vi "PH_uOPA_DelayController.set Control Status.vi"(0 "VI in":refnum<vi>, 2 "Control Status":T1, 5 "error in (no error)":errorcluster) -> (14 "VI out":refnum<vi>, 19 "error out":errorcluster)   [LabVIEW 2014, in "PH_uOPA_DelayController.lvlib"]
uses:
  PH_uOPA_DelayController.lvlib
  PH_uOPA_DelayController.Control Status.ctl
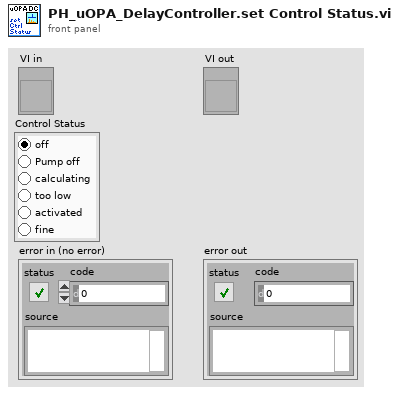
[diagram p1: front panel]
types:
  T1 = typedef "PH_uOPA_DelayController.lvlib/PH_uOPA_DelayController.Control Status.ctl" = enum32{"off", "Pump off", "calculating", "too low", "activated", "fine"}
  T2 = typedef "PH_uOPA_DelayController.lvlib/PH_uOPA_DelayController.i attribute.ctl" = cluster{"GUI Refs":cluster{"Current Pump Peak":refnum<vi>, "Current uOPA Peak":refnum<vi>, "Pump Peak":refnum<vi>, "uOPA Peak":refnum<vi>, "uOPA Target":refnum<vi>, "uOPA Limits [%]":refnum<vi>, "sample length":refnum<vi>, "Pump Target":refnum<vi>, "Pump Limit":refnum<vi>, "Pump running":refnum<vi>, "Feedback Control":refnum<vi>, "Control Status":refnum<vi>, "uOPA Mean":refnum<vi>, "Current uOPA Mean":refnum<vi>}, "uOPA Target":dbl, "uOPA Limits [%]":T3, "Sample Length":i32, "Initialize Mean":bool, "Pump Target":dbl, "Pump Limit [%]":dbl, "Feedback Control":bool, "Control Status":T1, "last Mean":dbl, "last direction":T4, "Axis Settings":T5, "Width while feedback":dbl}
  T3 = typedef "PH_uOPA_DelayController.lvlib/PH_uOPA_DelayController.Limit.ctl" = cluster{"low":dbl, "activate":dbl, "fine":dbl}
  T4 = typedef "PH_Stepmotor_BaseClass.lvlib/PH_Stepmotor_BaseClass.Axis Direction.ctl" = enum16{"forward", "backward"}
  T5 = typedef "PH_Stepmotor_BaseClass.lvlib/PH_Stepmotor_BaseClass.Axis Settings.ctl" = cluster{"Sign change":bool, "Width":dbl, "Calibration":dbl, "Unit":string, "Motor Type":T6, "Unit Width":string, "Unit CF":string}
  T6 = typedef "PH_Stepmotor_BaseClass.lvlib/PH_Stepmotor_BaseClass.Motor Type.ctl" = enum16{"Unspecific", "OWIS 49.120.2633", "OWIS 49.060.1033", "OWIS 43.040.2558", "Diamond Motion 2200 series", "OWIS 49.120.266B.MV6", "Calorimeter", "Linear Stage 1", "MICOS VT-80", "MICOS VT-80 S", "Standa Rotstage nt0.95A", "PUF RA 320.200", "PUF RA 800.200", "PUF RA 800.400", "PUF RA 400.50", "1324.nn.800.50", "1324.n9c.800.50", "1324.nn.320.200", "1324.nn.400.200", "1324.nn.800.200", "1324.nn.400.50", "1324.8c9c.800.50", "1324.8c9c.400.200"}
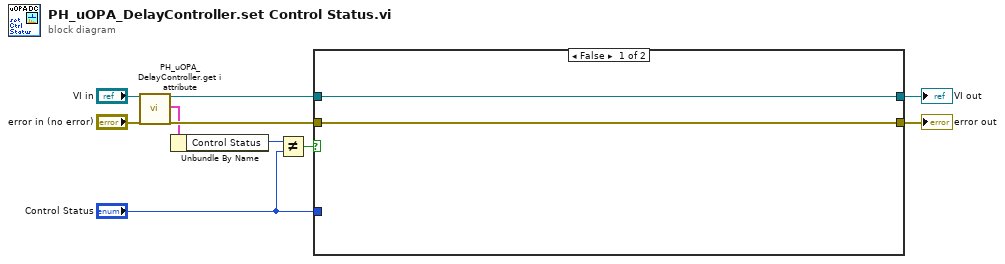
[diagram p0: block diagram]
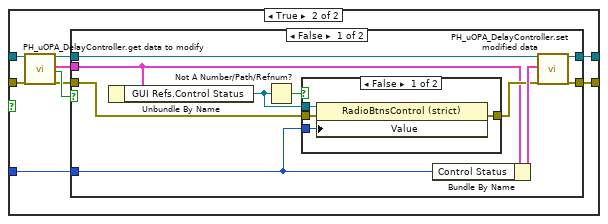
[diagram p2: hidden frame]
diagram:
  n1 = call "PH_uOPA_DelayController.get i attribute.vi"("i ref in"="VI in", "error in (no error)"="error in (no error)") -> ("i ref out"=w5:refnum<vi>, "i attribute"=w4:T2, "error out"=w7:errorcluster)  [unwired: 15 in]
  n2 = Unbundle By Name(w4) -> ("Control Status"=w3:T1)
  n3 = Not Equal?(x=w3, y="Control Status") -> (x != y?=w1:bool)
  n4 = case shown="False" w1 {
    tunnel: [w12 w19] -> w10
    tunnel: [w11 w16] -> w9
    tunnel: w7 -> [w11 w15]
    tunnel: w5 -> [w12 w14]
    tunnel: "Control Status" -> [_ w13]
    frame False {
    }
    frame True {
      n5 = call "PH_uOPA_DelayController.get data to modify.vi"("i ref in"=w14, "error in (no error)"=w15) -> ("i ref out"=w18:refnum<vi>, "i attribute"=w20:T2, "timed out"=w21:bool, "error out"=w17:errorcluster)  [unwired: 14 in]
      n6 = case shown="False" w21 {
        tunnel: [w31 w37] -> w16
        tunnel: w17 -> [w30 w37]
        tunnel: w18 -> [w29 w38]
        tunnel: [w28 w38] -> w19
        tunnel: w20 -> [w25 _]
        tunnel: w13 -> [w24 _]
        frame False {
          n7 = Unbundle By Name(w25) -> ("GUI Refs.Control Status"=w22:refnum<vi>)
          n8 = Not A Number/Path/Refnum?(number/path/refnum=w22) -> (NaN/Path/Refnum?=w23:bool)
          n9 = case shown="False" w23 {
            tunnel: w30 -> [w35 w36]
            tunnel: [w34 w36] -> w26
            tunnel: w22 -> [w33 _]
            tunnel: w24 -> [w32 _]
            frame False {
              n10 = property class="RadioBtnsControl (strict)"(reference=w33, error in=w35, "Value"=w32) -> (error out=w34:errorcluster)  [unwired: 1 out]
            }
            frame True {
            }
          }
          n11 = Bundle By Name(cluster=w25, "Control Status"=w24) -> (w27:T2)
          n12 = call "PH_uOPA_DelayController.set modified data.vi"("i ref in"=w29, "i attribute"=w27, "error in (no error)"=w26) -> ("i ref out"=w28:refnum<vi>, "error out"=w31:errorcluster)  [unwired: 15 in]
        }
        frame True {
        }
      }
    }
  }
  "VI out" <- w10
  "error out" <- w9
